vi "Digilent Basic IO Shield - OLED Config.vi"(8 "Error In":errorcluster, 11 "LINX Resource":T1) -> (0 "Error Out":errorcluster, 3 "LINX Resource":T1)   [LabVIEW 2013, in "LVH-LINX.lvlib" / "SSD1306.lvlib"]
uses:
  <vilib>/LabVIEW Hacker/LINX/Public/Sensors/Display/SSD1306/SSD1306.lvlib
  <vilib>/LabVIEW Hacker/LINX/Private/Type Defs/LINX Ref.ctl
  <vilib>/LabVIEW Hacker/LINX/Private/Type Defs/Platform.ctl
  <vilib>/LabVIEW Hacker/LINX/Private/Type Defs/Interface.ctl
  <vilib>/LabVIEW Hacker/LINX/Private/Device/Type Defs/LINX Device Config.ctl
  <vilib>/LabVIEW Hacker/LINX/Private/Device/Type Defs/TCP Config.ctl
  <vilib>/LabVIEW Hacker/LINX/Private/Type Defs/Device Family.ctl
  <vilib>/LabVIEW Hacker/LINX/Public/Sensors/Display/SSD1306/Private/SSD1306 Config.ctl
  <vilib>/LabVIEW Hacker/LINX/LVH-LINX.lvlib
  <vilib>/LabVIEW Hacker/LINX/Private/Device/Device.lvlib
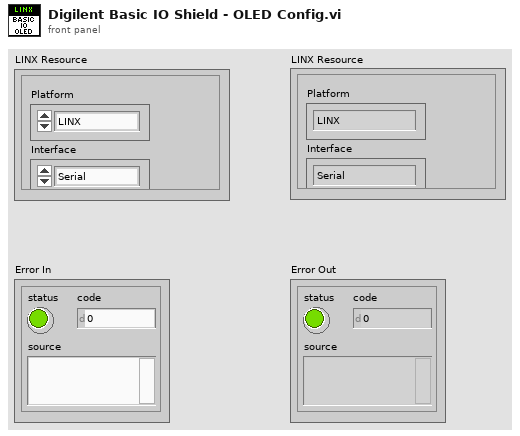
[diagram p1: front panel]
types:
  T1 = typedef "LVH-LINX.lvlib/LINX Ref.ctl" = cluster{"Platform":T2, "Interface":T3, "LINX Device Config":T4}
  T2 = typedef "LVH-LINX.lvlib/Platform.ctl" = enum16{"LINX", "myRIO"}
  T3 = typedef "LVH-LINX.lvlib/Interface.ctl" = enum16{"Serial", "TCP"}
  T4 = typedef "LVH-LINX.lvlib/Device.lvlib/LINX Device Config.ctl" = cluster{"Interface":T3, "COM Port":refnum<visa-resource-name>, "TCP Configuration":T5, "Device Family":T6, "Device ID":u8, "Device Name":string, "TCP Ref":refnum<k5>}
  T5 = typedef "LVH-LINX.lvlib/Device.lvlib/TCP Config.ctl" = cluster{"IP Address":string, "Port":u16}
  T6 = typedef "LVH-LINX.lvlib/Device Family.ctl" = enum8{"National Instruments", "Digilent", "Arduino"}
  T7 = typedef "LVH-LINX.lvlib/SSD1306.lvlib/SSD1306 Config.ctl" = cluster{"SPI Channel (0)":u8, "VDD Channel":u8, "VBAT Channel":u8, "RESET Channel":u8, "DC Channel":u8, "SPI CS (3)":u8}
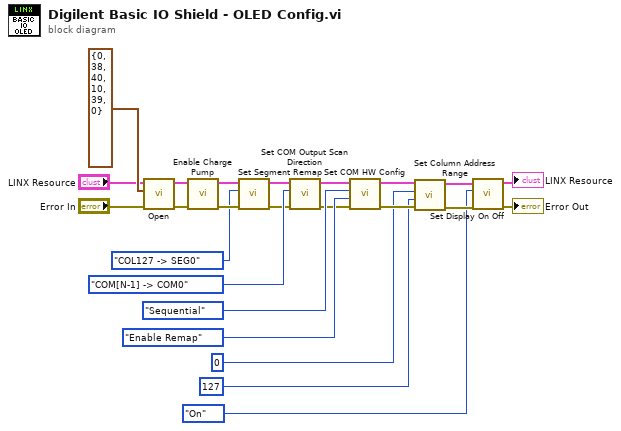
[diagram p0: block diagram]
diagram:
  n1 = call <vilib>:"Open.vi"("Error In"="Error In", "SSD1306 Channels"=T7 {"SPI Channel (0)"=0, "VDD Channel"=38, "VBAT Channel"=40, "RESET Channel"=10, "DC Channel"=39, "SPI CS (3)"=0}, "LINX Resource"="LINX Resource") -> ("Error Out"=w22:errorcluster, "LINX Resource"=w23:T1)  [unwired: 7 in]
  n2 = call <vilib>:"Enable Charge Pump.vi"("Error In"=w22, "LINX Resource"=w23) -> ("Error Out"=w21:errorcluster, "LINX Resource"=w20:T1)  [unwired: 8 in]
  n3 = call <vilib>:"Set Segment Remap.vi"("Error In"=w21, "Segment Remap"=enum8{"COL 0 -> SEG0", "COL127 -> SEG0"}."COL127 -> SEG0", "LINX Resource"=w20) -> ("Error Out"=w14:errorcluster, "LINX Resource"=w15:T1)  [unwired: 7 in]
  n4 = call <vilib>:"Set COM Output Scan Direction.vi"("Error In"=w14, "COM Direction"=enum8{"COM0 -> COM[N-1]", "COM[N-1] -> COM0"}."COM[N-1] -> COM0", "LINX Resource"=w15) -> ("Error Out"=w12:errorcluster, "LINX Resource"=w13:T1)  [unwired: 7 in]
  n5 = call <vilib>:"Set COM HW Config.vi"("Error In"=w12, "COM Left/Right Remap"=enum8{"Disable Remap", "Enable Remap"}."Enable Remap", "COM Pin Config"=enum8{"Sequential", "Alternative"}."Sequential", "LINX Resource"=w13) -> ("Error Out"=w11:errorcluster, "LINX Resource"=w10:T1)  [unwired: 6 in]
  n6 = call <vilib>:"Set Column Address Range.vi"("Error In"=w11, "Column End Address"=u8 127 ("Column Start Address"), "Column Start Address"=u8 0, "LINX Resource 2"=w10) -> ("Error Out"=w7:errorcluster, "LINX Resource"=w6:T1)  [unwired: 6 in]
  n7 = call <vilib>:"Set Display On Off.vi"("Error In"=w7, "Display On/Off"=enum8{"Off", "On"}."On", "LINX Resource 2"=w6) -> ("Error Out"=→"Error Out":errorcluster, "LINX Resource"=→"LINX Resource":T1)  [unwired: 7 in]
